vi "SPconTrig.vi"(6 "Trigger":T2 {"Coupling" items=["DC 1 MOhm", "AC 1 MOhm", "DC 50 Ohm", "AC 50 Ohm"]; "Slope" items=["Positive", "Negative"]; "Level" format="%.2f"; "Source" items=["Chan 1", "External"]}, 8 "error in":errorcluster, 9 "adq_num":i32, 10 "adq_cu_ptr":refnum<k24>, 11 "ADQAPI Ref":refnum<k24>) -> (0 "error out":errorcluster, 2 "adq_cu_ptr (out)":refnum<k24>, 3 "ADQAPI Ref (out)":refnum<k24>)   [LabVIEW 2022 SP3]
uses:
  C:/Windows/System32/ADQAPI_dotNet_helper.dll
  ADQTriggerMode.ctl
  ADQClockSource.ctl
  ADQTriggerEdge.ctl
  ADQAPI.lvlib
panel:
  out "Status":T1
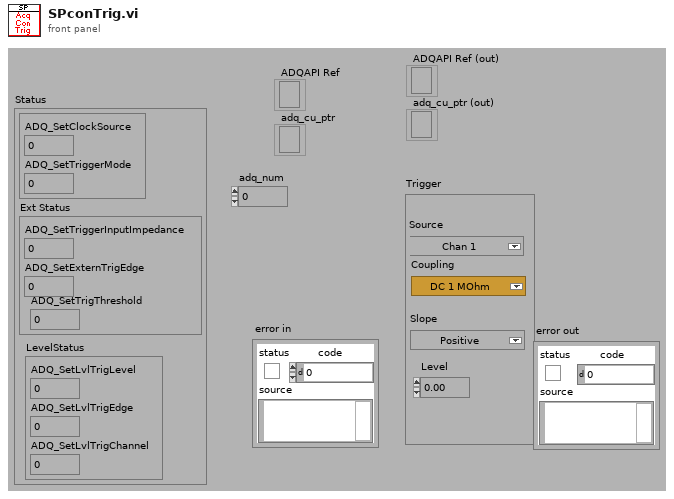
[diagram p1: front panel]
types:
  T1 = cluster{cluster{"ADQ_SetClockSource":i32, "ADQ_SetTriggerMode":i32}, "Ext Status":cluster{"ADQ_SetTriggerInputImpedance":i32, "ADQ_SetExternTrigEdge":u32, "ADQ_SetTrigThreshold":i32}, "LevelStatus":cluster{"ADQ_SetLvlTrigLevel":i32, "ADQ_SetLvlTrigEdge":i32, "ADQ_SetLvlTrigChannel":i32}}
  T2 = cluster{"Source":u16, "Coupling":u16, "Slope":u16, "Level":dbl}
  T3 = typedef "ADQAPI.lvlib/ADQClockSource.ctl" = enum16{"ADQ_CLOCK_INT_INTREF", "ADQ_CLOCK_INT_EXTREF", "ADQ_CLOCK_EXT", "ADQ_CLOCK_INT_PXIREF"}
  T4 = typedef "ADQAPI.lvlib/ADQTriggerMode.ctl" = i32
  T5 = typedef "ADQAPI.lvlib/ADQTriggerEdge.ctl" = enum16{"ADQ_TRIGGER_FALLING_EDGE", "ADQ_TRIGGER_RISING_EDGE"}
  T6 = cluster{"ADQ_SetTriggerInputImpedance":i32, "ADQ_SetExternTrigEdge":u32, "ADQ_SetExtTrigThreshold":u32}
  T7 = cluster{"ADQ_SetLvlTrigLevel":i32, "ADQ_SetLvlTrigEdge":i32, "ADQ_SetLvlTrigChannel":i32}
  T8 = cluster{"ADQ_SetClockSource":i32, "ADQ_SetTriggerMode":i32}
  T9 = cluster{cluster{"ADQ_SetClockSource":i32, "ADQ_SetTriggerMode":i32}, cluster{"ADQ_SetTriggerInputImpedance":i32, "ADQ_SetExternTrigEdge":u32, "ADQ_SetExtTrigThreshold":u32}, cluster{"ADQ_SetLvlTrigLevel":i32, "ADQ_SetLvlTrigEdge":i32, "ADQ_SetLvlTrigChannel":i32}}
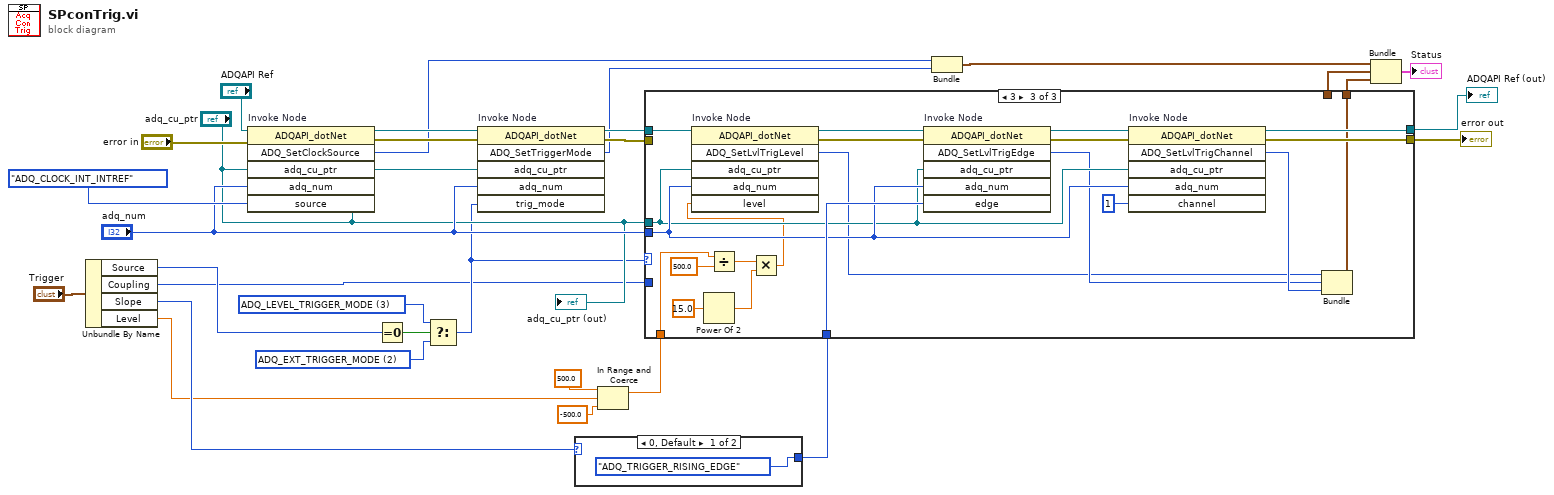
[diagram p0: block diagram]
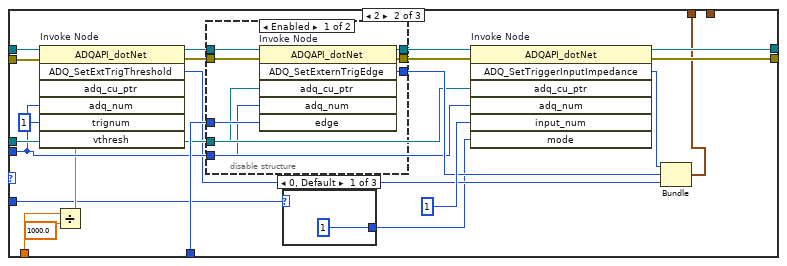
[diagram p3: hidden frame]
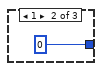
[diagram p4: hidden frame]
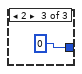
[diagram p5: hidden frame]
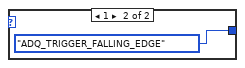
[diagram p7: hidden frame]
diagram:
  w26 = T4 3 items=["ADQ_SW_TRIGGER_MODE"=1, "ADQ_EXT_TRIGGER_MODE"=2, "ADQ_LEVEL_TRIGGER_MODE"=3, "ADQ_INTERNAL_TRIGGER_MODE"=4] ("ADQTriggerMode")
  w27 = T4 2 items=["ADQ_SW_TRIGGER_MODE"=1, "ADQ_EXT_TRIGGER_MODE"=2, "ADQ_LEVEL_TRIGGER_MODE"=3, "ADQ_INTERNAL_TRIGGER_MODE"=4] ("ADQTriggerMode")
  n1 = Unbundle By Name("Trigger") -> ("Source"=w25:u16, "Coupling"=w1:u16, "Slope"=w28:u16, "Level"=w4:dbl)
  n2 = invoke on="Invoke Node" class="ADQAPI_dotNet" method="ADQ_SetClockSource"(reference="ADQAPI Ref", error in="error in", "adq_cu_ptr"="adq_cu_ptr", "adq_num"="adq_num", "source"=ADQClockSource."ADQ_CLOCK_INT_INTREF" ("cllockSource")) -> (reference out=w19:refnum<k24>, error out=w17:errorcluster, "ADQ_SetClockSource"=w10:i32)  [unwired: 1 in, 3 out]
  n3 = Equal To 0?(x=w25) -> (x = 0?=w29:bool)
  n4 = Select(t=w26, s=w29, f=w27) -> (s? t:f=w13:T4)
  n5 = invoke on="Invoke Node" class="ADQAPI_dotNet" method="ADQ_SetTriggerMode"(reference=w19, error in=w17, "adq_cu_ptr"="adq_cu_ptr", "adq_num"="adq_num", "trig_mode"=w13) -> (reference out=w18:refnum<k24>, error out=w12:errorcluster, "ADQ_SetTriggerMode"=w11:i32)  [unwired: 1 in, 3 out]
  n6 = case shown="0, Default" w28 {
    tunnel: [ADQTriggerEdge."ADQ_TRIGGER_RISING_EDGE" ("ADQTriggerEdge") ADQTriggerEdge."ADQ_TRIGGER_FALLING_EDGE" ("ADQTriggerEdge")] -> w22
    frame 0, Default {
    }
    frame 1 {
    }
  }
  n7 = In Range and Coerce(upper limit=500.0, x=w4, lower limit=-500.0 ("upper limit")) -> (coerced(x)=w2:dbl)  [unwired: 1 out]
  n8 = case shown="3" w13 {
    tunnel: w22 -> [_ w56 w90]
    tunnel: "adq_num" -> [_ w42 w89]
    tunnel: w18 -> [w34 w47 w88]
    tunnel: [w33 w53 w83] -> w16
    tunnel: "adq_cu_ptr" -> [_ w43 w82]
    tunnel: [w34 w52 w81] -> w14
    tunnel: w12 -> [w33 w46 _]
    tunnel: [_ _ w77] -> w7
    tunnel: [_ w48 _] -> w6
    tunnel: w2 -> [_ w39 w73]
    tunnel: w1 -> [_ w36 _]
    frame 0, Default {
    }
    frame 2 {
      n9 = Divide(x=w39, y=1000.0) -> (x/y=w37:dbl)
      n10 = invoke on="Invoke Node" class="ADQAPI_dotNet" method="ADQ_SetExtTrigThreshold"(reference=w47, error in=w46, "adq_cu_ptr"=w43, "adq_num"=w42, "trignum"=u32 1, "vthresh"=w37) -> (reference out=w45:refnum<k24>, error out=w44:errorcluster, "ADQ_SetExtTrigThreshold"=w41:u32)  [unwired: 1 in, 4 out]
      n11 = disable-structure shown="Enabled" {
        disable-tunnel: w56 -> [w67 _]
        disable-tunnel: w42 -> [w66 _]
        disable-tunnel: [w65 w69] -> w55
        disable-tunnel: [w64 w68] -> w54
        disable-tunnel: w43 -> [w63 _]
        disable-tunnel: w45 -> [w62 w69]
        disable-tunnel: w44 -> [w61 w68]
        disable-tunnel: [w60 _] -> w50
        frame Enabled {
          n12 = invoke on="Invoke Node" class="ADQAPI_dotNet" method="ADQ_SetExternTrigEdge"(reference=w62, error in=w61, "adq_cu_ptr"=w63, "adq_num"=w66, "edge"=w67) -> (reference out=w65:refnum<k24>, error out=w64:errorcluster, "ADQ_SetExternTrigEdge"=w60:u32)  [unwired: 1 in, 3 out]
        }
        frame Disabled {
        }
      }
      n13 = case shown="0, Default" w36 {
        tunnel: [1 0 0] -> w35
        frame 0, Default {
        }
        frame 1 {
        }
        frame 2 {
        }
      }
      n14 = invoke on="Invoke Node" class="ADQAPI_dotNet" method="ADQ_SetTriggerInputImpedance"(reference=w55, error in=w54, "adq_cu_ptr"=w43, "adq_num"=w42, "input_num"=1, "mode"=w35) -> (reference out=w52:refnum<k24>, error out=w53:errorcluster, "ADQ_SetTriggerInputImpedance"=w49:i32)  [unwired: 1 in, 4 out]
      n15 = Bundle("ADQ_SetTriggerInputImpedance"=w49, "ADQ_SetExternTrigEdge"=w50, "ADQ_SetExtTrigThreshold"=w41) -> (w48:T6)  [unwired: 1 in]
    }
    frame 3 {
      n16 = Power Of 2(x=15.0) -> (2^x=w71:dbl)
      n17 = Divide(x=w73, y=500.0) -> (x/y=w72:dbl)
      n18 = Multiply(x=w72, y=w71) -> (x*y=w70:dbl)
      n19 = invoke on="Invoke Node" class="ADQAPI_dotNet" method="ADQ_SetLvlTrigLevel"(reference=w88, "adq_cu_ptr"=w82, "adq_num"=w89, "level"=w70) -> (reference out=w87:refnum<k24>, error out=w86:errorcluster, "ADQ_SetLvlTrigLevel"=w78:i32)  [unwired: 2 in, 3 out]
      n20 = invoke on="Invoke Node" class="ADQAPI_dotNet" method="ADQ_SetLvlTrigEdge"(reference=w87, error in=w86, "adq_cu_ptr"=w82, "adq_num"=w89, "edge"=w90) -> (reference out=w85:refnum<k24>, error out=w84:errorcluster, "ADQ_SetLvlTrigEdge"=w79:i32)  [unwired: 1 in, 3 out]
      n21 = invoke on="Invoke Node" class="ADQAPI_dotNet" method="ADQ_SetLvlTrigChannel"(reference=w85, error in=w84, "adq_cu_ptr"=w82, "adq_num"=w89, "channel"=1) -> (reference out=w81:refnum<k24>, error out=w83:errorcluster, "ADQ_SetLvlTrigChannel"=w80:i32)  [unwired: 1 in, 3 out]
      n22 = Bundle("ADQ_SetLvlTrigLevel"=w78, "ADQ_SetLvlTrigEdge"=w79, "ADQ_SetLvlTrigChannel"=w80) -> (w77:T7)  [unwired: 1 in]
    }
  }
  "error out" <- w16
  "ADQAPI Ref (out)" <- w14
  n23 = Bundle("ADQ_SetClockSource"=w10, "ADQ_SetTriggerMode"=w11) -> (w9:T8)  [unwired: 1 in]
  n24 = Bundle(w9, w6, w7) -> (→"Status":T9)  [unwired: 1 in]
  "adq_cu_ptr (out)" <- "adq_cu_ptr"
